vi "FFT Conversion.vi"(2 "Number of Channels":u32, 3 "Frame Rate":dbl, 4 "input array":dbl[](array[numeric])) -> (0 "X scale factor":dbl, 1 "FFT":dbl[](array[numeric]))   [LabVIEW 2010]
uses:
  <vilib>/Analysis/4window.llb/Hanning Window (DBL).vi
  <vilib>/Analysis/2dsp.llb/Real FFT.vi
  <vilib>/Analysis/NI_AALPro.lvlib
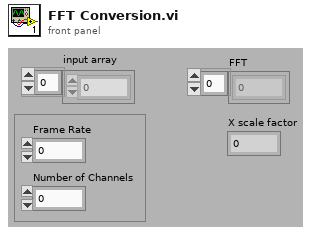
[diagram p1: front panel]
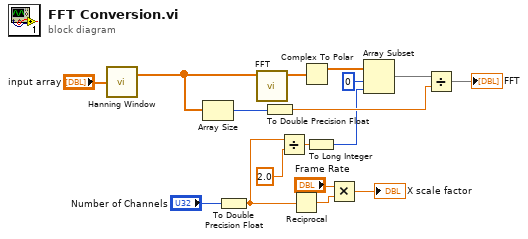
[diagram p0: block diagram]
diagram:
  n1 = call-poly <vilib>:"Hanning Window.vi"("X"="input array") -> ("Windowed X"=w12:dbl[])  [unwired: 1 out]
  n2 = Array Size(array=w12) -> (size(s)=w14:i32)
  n3 = To Double Precision Float(number="Number of Channels") -> (double precision float=w8:dbl)
  n4 = call-poly <vilib>:"FFT.vi"("X"=w12) -> ("FFT {X}"=w15:cdb[])  [unwired: 9 in, 1 out]
  n5 = To Double Precision Float(number=w14) -> (double precision float=w13:dbl)
  n6 = Divide(x=w8, y=2.0) -> (x/y=w7:dbl)
  n7 = Reciprocal(x=w8) -> (1/x=w5:dbl)
  n8 = Complex To Polar(r * e^(i*theta)=w15) -> (r=w16:dbl[])  [unwired: 1 out]
  n9 = To Long Integer(number=w7) -> (32bit integer=w4:i32)
  n10 = Multiply(x="Frame Rate", y=w5) -> (x*y=→"X scale factor":dbl)
  n11 = Array Subset(array=w16, index=0 ("length"), length=w4) -> (w17:dbl[])
  n12 = Divide(x=w17, y=w13) -> (x/y=→"FFT":dbl[])
